vi "Write TDMS File.vi"(7 "channel name(s)":string[](array[string])=["VoltageFB", "CurrentFB"], 8 "error in (no error)":errorcluster, 9 "TDMS Enabled":bool, 10 "Wfm data (NChanNSamp)":waveform(dbl)[](array[waveform]), 11 "tdms ref":refnum<k34>) -> (0 "error out":errorcluster, 3 "tdms ref out":refnum<k34>)   [LabVIEW 2017, in "LogEngine.lvclass"]
doc: "Developed by Kevin Thompson\nkevin@thompsonengineering.net\n\nCopyright 2018-2020\nThompson Engineering, LLC"
uses:
  LogEngine.lvclass
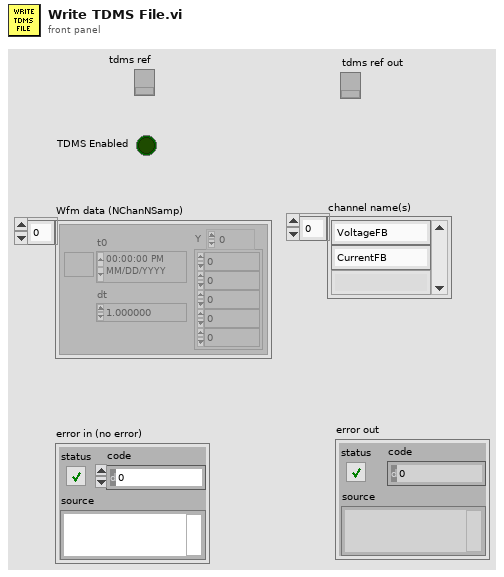
[diagram p1: front panel]
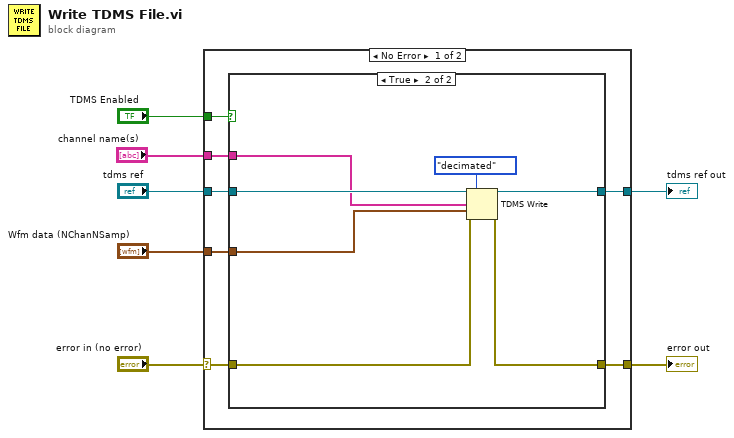
[diagram p0: block diagram]
diagram:
  n1 = case shown="No Error" "error in (no error)" {
    selector: "error in (no error)" -> [w9 w24]
    tunnel: "tdms ref" -> [w14 w25]
    tunnel: "Wfm data (NChanNSamp)" -> [w13 _]
    tunnel: [w12 w24] -> w5
    tunnel: [w11 w25] -> w4
    tunnel: "TDMS Enabled" -> [w10 _]
    tunnel: "channel name(s)" -> [w8 _]
    frame No Error {
      n2 = case shown="True" w10 {
        tunnel: w14 -> [w16 w23]
        tunnel: w13 -> [_ w22]
        tunnel: w9 -> [w15 w20]
        tunnel: [w15 w19] -> w12
        tunnel: [w16 w18] -> w11
        tunnel: w8 -> [_ w17]
        frame False {
        }
        frame True {
          n3 = TDMS Write(0:w23, 1:enum16{"decimated", "interleaved"}."decimated" ("data layout (0:decimated)"), 7:w17, 9:w22, 11:w20) -> (4:w18:refnum<k34>, 15:w19:errorcluster)  [unwired: 1 in, 2 out]
        }
      }
    }
    frame Error {
    }
  }
  "error out" <- w5
  "tdms ref out" <- w4
